vi "whileState.vi"(8 "error in (no error)":errorcluster, 11 "shuttingDown in":refnum<class "shuttingDown.lvclass">) -> (0 "error out":errorcluster, 1 "Done?":bool, 2 "next state":refnum<class "state.lvclass">, 3 "shuttingDown out":refnum<class "shuttingDown.lvclass">)   [LabVIEW 2020, in "eos.lvlib" / "shuttingDown.lvclass"]
uses:
  shuttingDown.lvclass
  interfaces/state/state.lvclass
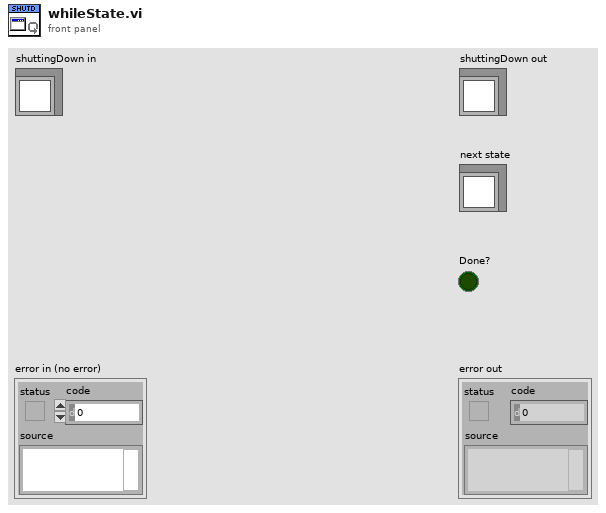
[diagram p1: front panel]
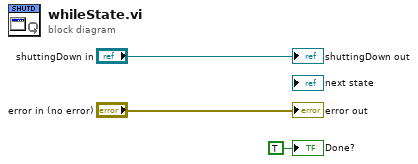
[diagram p0: block diagram]
diagram:
  "error out" <- "error in (no error)"
  "shuttingDown out" <- "shuttingDown in"
  "Done?" <- TRUE ("Done?")
